vi "Two 32-bit Port Digital Output.vi"(2 "Packet":u64, 4 "Two 32-bit DO Ports":T1={"32-Bit DO Port0"="Chassis2/Mod4/DIO31:0", "32-Bit DO Port1"="Chassis2/Mod4/DIO31:0"}) -> ()   [LabVIEW 2010]
uses:
  <vilib>/eio/EIONode/EIONode.xnode
  <vilib>/rvi/eio/nirviEIOImplementation/nirviEIOImplementation.xnode
  <vilib>/rvi/eio/common/nirviEmuClasses.ctl
  <vilib>/rvi/eio/common/nirviEmuTemplateMethod_noerrors.vi
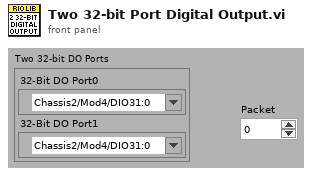
[diagram p1: front panel]
types:
  T1 = cluster{"32-Bit DO Port0":refnum<k21>, "32-Bit DO Port1":refnum<k21>}
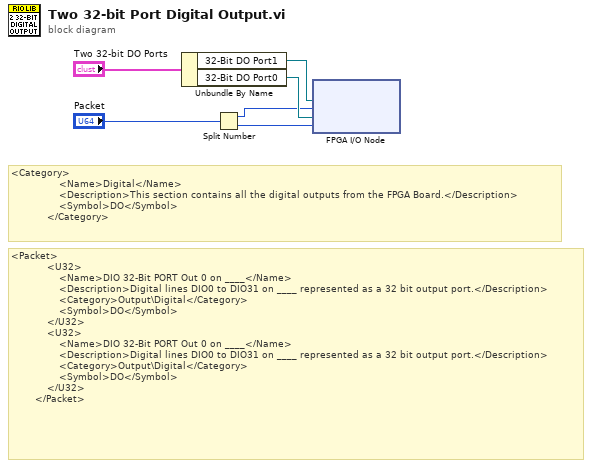
[diagram p0: block diagram]
diagram:
  # "<Packet>\n            <U32>\n                <Name>DIO 32-Bit PORT Out 0 on ____</Name>\n                <Description>Digital lines DIO0 to DIO31 on ____ represented as a 32 bit output port.</Description>\n                <Category>Output\\Digital</Category>\n                <Symbol>DO</Symbol>\n            </U32>\n            <U32>\n                <Name>DIO 32-Bit PORT Out 0 on ____</Name>\n                <Description>Digital lines DIO0 to DIO31 on ____ represented as a 32 bit output port.</Description>\n                <Category>Output\\Digital</Category>\n                <Symbol>DO</Symbol>\n            </U32>\n        </Packet>"
  # "<Category>\n                <Name>Digital</Name>\n                <Description>This section contains all the digital outputs from the FPGA Board.</Description>\n                <Symbol>DO</Symbol>\n            </Category>"
  n1 = Unbundle By Name("Two 32-bit DO Ports") -> ("32-Bit DO Port1"=w2:refnum<k21>, "32-Bit DO Port0"=w3:refnum<k21>)
  n2 = Split Number(x="Packet") -> (hi(x)=w1:u32, lo(x)=w5:u32)
  n3 = xnode "FPGA I/O Node"("I/O Item"=w1, "I/O Item"=w5, "FPGA I/O In"=w2, "FPGA I/O In"=w3) -> ()  [unwired: 2 out]
